vi "Configure Offset and Limits (Spectrum Emission Mask - Relative and Absolute Limits).vi"(0 "VISA resource name":refnum<visa-resource-name>, 1 "Manual Absolute Stop List":dbl[](array[numeric])=[-14.0, -14.0, -14.0, -14.0, -14.0] format="%#.6g", 3 "Manual Relative Stop List":dbl[](array[numeric])=[-30.0, -30.0, -30.0, -30.0, -30.0] format="%#.6g", 5 "Absolute Start List":dbl[](array[numeric])=[-14.0, -14.0, -14.0, -14.0, -14.0] format="%#.6g", 9 "Relative Start List":dbl[](array[numeric])=[-30.0, -30.0, -30.0, -30.0, -30.0] format="%#.6g", 11 "error in (no error)":errorcluster, 12 "Fail Mask List":i32[](array[ring])=[0, 0, 0, 0, 0] items=["Absolute", "Absolute And Relative", "Absolute Or Relative", "Relative"]) -> (4 "VISA resource name out":refnum<visa-resource-name>, 15 "error out":errorcluster)   [LabVIEW 2022 SP3, in "Agilent N934X Series.lvlib"]
doc: "Configures the relative and absolute settings under offsets and limits of SEM measurement type.\n\nNote:\nThis VI is only applicable for N9321C, N9322C, N9323C, N9324C models."
uses:
  <instrlib>/Agilent N934X Series/Agilent N934X Series.lvlib
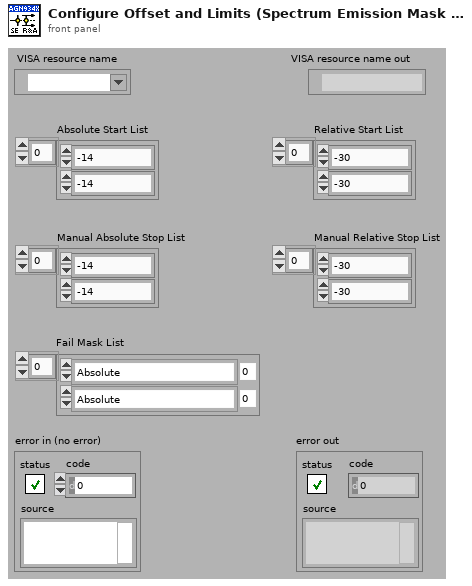
[diagram p1: front panel]
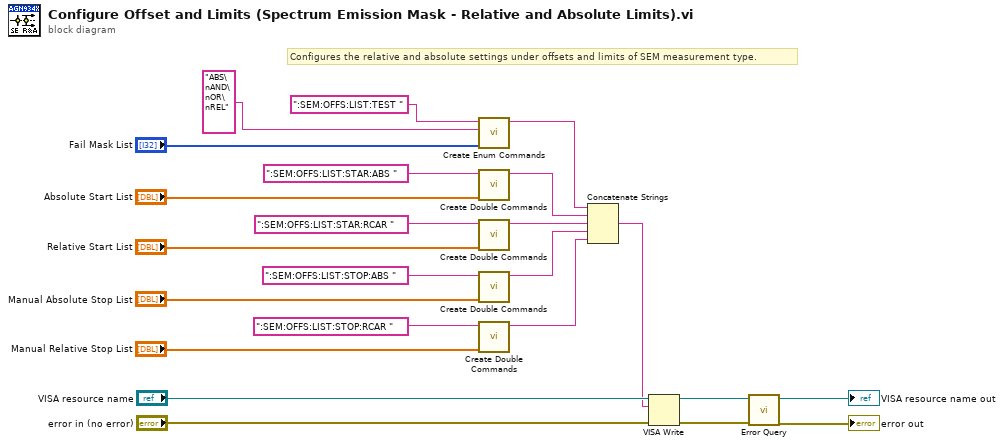
[diagram p0: block diagram]
diagram:
  # "Configures the relative and absolute settings under offsets and limits of SEM measurement type."
  n1 = call <instrlib>:"Create Enum Commands.vi"("Enum Values"="Fail Mask List", "Multi-line Text"="ABS\nAND\nOR\nREL" ("multi-line string"), "Commands"=":SEM:OFFS:LIST:TEST " ("format string")) -> ("Result"=w17:string)  [unwired: 8 in]
  n2 = call <instrlib>:"Create Double Commands.vi"("Double Values"="Absolute Start List", "Commands"=":SEM:OFFS:LIST:STAR:ABS " ("format string")) -> ("Result"=w11:string)  [unwired: 9 in]
  n3 = call <instrlib>:"Create Double Commands.vi"("Double Values"="Relative Start List", "Commands"=":SEM:OFFS:LIST:STAR:RCAR " ("format string")) -> ("Result"=w8:string)  [unwired: 9 in]
  n4 = call <instrlib>:"Create Double Commands.vi"("Double Values"="Manual Absolute Stop List", "Commands"=":SEM:OFFS:LIST:STOP:ABS " ("format string")) -> ("Result"=w5:string)  [unwired: 9 in]
  n5 = call <instrlib>:"Create Double Commands.vi"("Double Values"="Manual Relative Stop List", "Commands"=":SEM:OFFS:LIST:STOP:RCAR " ("format string")) -> ("Result"=w2:string)  [unwired: 9 in]
  n6 = Concatenate Strings(w17, w11, w8, w5, w2) -> (w1:string)
  n7 = VISA Write(VISA resource name="VISA resource name", write buffer=w1, error in (no error)="error in (no error)") -> (VISA resource name out=w21:refnum<visa-resource-name>, error out=w20:errorcluster)  [unwired: 1 out]
  n8 = call <instrlib>:"Error Query.vi"("error in (no error)"=w20, "VISA resource name"=w21) -> ("error out"=→"error out":errorcluster, "VISA resource name out"=→"VISA resource name out":refnum<visa-resource-name>)  [unwired: 6 in, 2 out]
